vi "Recolor.vi"(11 "Array in":refnum<vi>) -> (2 "Files":T1[](array[typedef]))   [LabVIEW 2022 SP3]
uses:
  Curtin1_Label.ctl
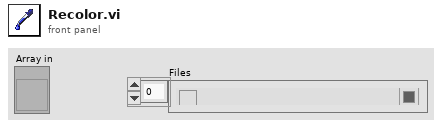
[diagram p1: front panel]
types:
  T1 = typedef "Curtin1_Label.ctl" = cluster{"Show?":bool, "Name":string, "Color":u32, "Path":path, "Show Notes":bool}
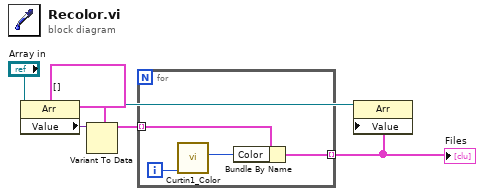
[diagram p0: block diagram]
diagram:
  n1 = property class="Arr"(reference="Array in") -> (reference out=w2:refnum<vi>, "Value"=w4:variant)  [unwired: 1 in, 1 out]
  n2 = Variant To Data(type=T1[] [] ("Files"), Variant=w4) -> (data=w6:T1[])  [unwired: 1 in, 1 out]
  n3 = for {
    tunnel: w6 -> [w10] mode=indexing
    tunnel: [w7] -> w1 mode=indexing
    i -> [w9]
    n4 = call "Curtin1_Color.vi"("Offset"=w9) -> ("New color"=w8:u32)  [unwired: 9 in, 1 out]
    n5 = Bundle By Name(cluster=w10, "Color"=w8) -> (w7:T1)
  }
  "Files" <- w1
  n6 = property class="Arr"(reference=w2, "Value"=w1) -> ()  [unwired: 1 in, 2 out]
